vi "Read Setpoint.vi"(8 "error in (no error)":errorcluster, 11 "MFC in":refnum<class "Control.lvclass">) -> (0 "error out":errorcluster, 2 "Setpoint 1":refnum<vi>, 3 "MFC out":refnum<class "Control.lvclass">)   [LabVIEW 2013, in "Control.lvib.lvlib" / "Control.lvclass"]
uses:
  Control.lvclass
  Control.lvclass/Control.ctl
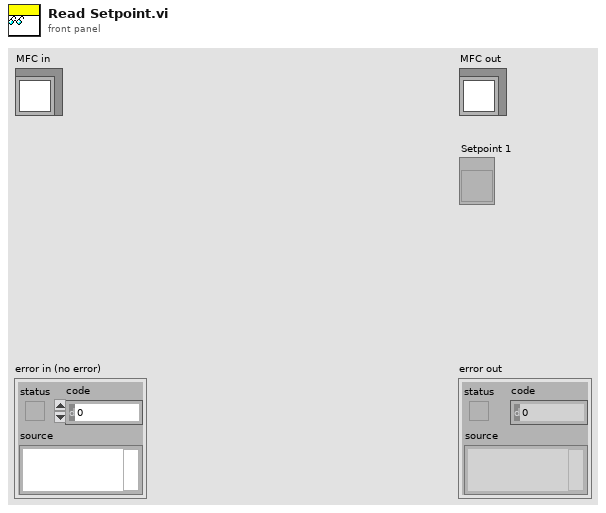
[diagram p1: front panel]
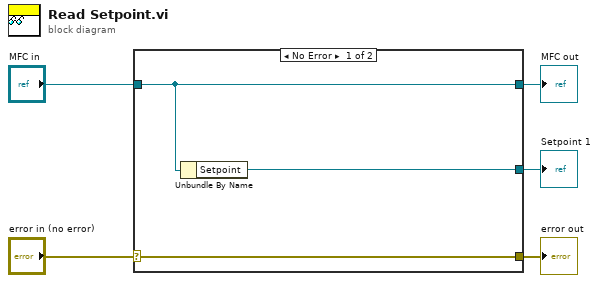
[diagram p0: block diagram]
diagram:
  n1 = case shown="No Error" "error in (no error)" {
    selector: "error in (no error)" -> [w8 w9]
    tunnel: [w8 w9] -> w4
    tunnel: [w7 w10] -> w2
    tunnel: "MFC in" -> [w7 w10]
    tunnel: [w6 _] -> w1
    frame No Error {
      n2 = Unbundle By Name(w7) -> ("Setpoint"=w6:refnum<vi>)
    }
    frame Error {
    }
  }
  "error out" <- w4
  "MFC out" <- w2
  "Setpoint 1" <- w1
